vi "Get Neuron Offset.vi"(11 "Grid in":refnum<class "Grid.lvclass">) -> (2 "Neurons Offset Index":i32[](array[numeric]), 3 "Grid out":refnum<class "Grid.lvclass">)   [LabVIEW 2016, in "Grid.lvclass"]
doc: "This Vi returns an array wth the offsets of neurons"
uses:
  Grid.lvclass
  Grid.lvclass/Grid.ctl
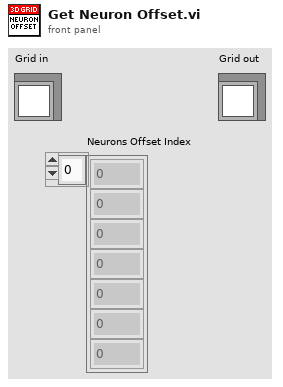
[diagram p1: front panel]
types:
  T1 = typedef "Neuron Info.ctl" = cluster{"N":i32, "Radius":dbl, "Type":T2, "Color":u32}[]
  T2 = typedef "Type of Neuron.ctl" = enum16{"MF", "BA", "GO", "GC", "PC", "LU", "Glia (Dummy)"}
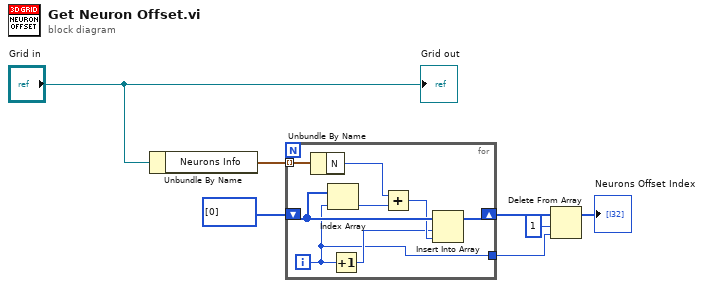
[diagram p0: block diagram]
diagram:
  n1 = Unbundle By Name("Grid in") -> ("Neurons Info"=w6:T1)
  n2 = for {
    tunnel: w6 -> [w15] mode=indexing
    shift-right: [w13] -> w4
    shift-left: i32[] [0] -> [w12]
    tunnel: [w8] -> w1
    i -> [w8]
    n3 = Unbundle By Name(w15) -> ("N"=w14:i32)
    n4 = Index Array(array=w12, index=w8) -> (element=w11:i32)
    n5 = Increment(x=w8) -> (x+1=w9:i32)
    n6 = Add(x=w14, y=w11) -> (x+y=w10:i32)
    n7 = Insert Into Array(array=w12, index=w9, new element=w10) -> (w13:i32[])
  }
  n8 = Delete From Array(array=w4, length=1, index=w1) -> (array with subset deleted=→"Neurons Offset Index":i32[])  [unwired: 1 out]
  "Grid out" <- "Grid in"
